vi "Get IO Names.vi"(8 "error in (no error)":errorcluster, 11 "Module in":refnum<class "Module.lvclass">) -> (0 "error out":errorcluster, 2 "IO Names":string[](array[string]), 3 "Module out":refnum<class "Module.lvclass">)   [LabVIEW 2019, in "Module.lvclass"]
uses:
  Module.lvclass
  Module.lvclass/Module.ctl
  Signal/Signal/Read IO Name.vi
  Signal/Signal/Signal.lvclass
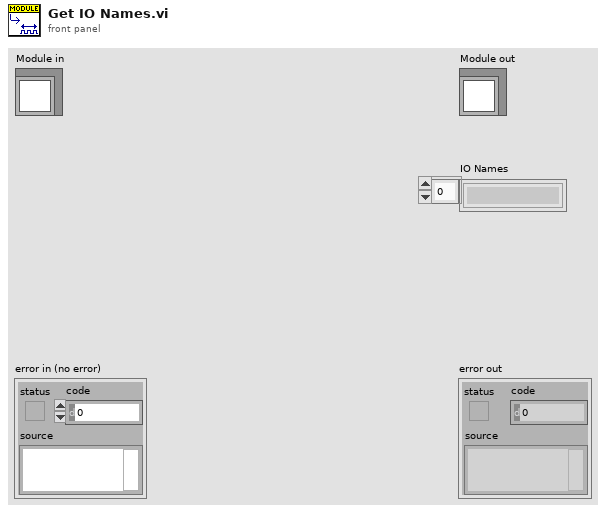
[diagram p1: front panel]
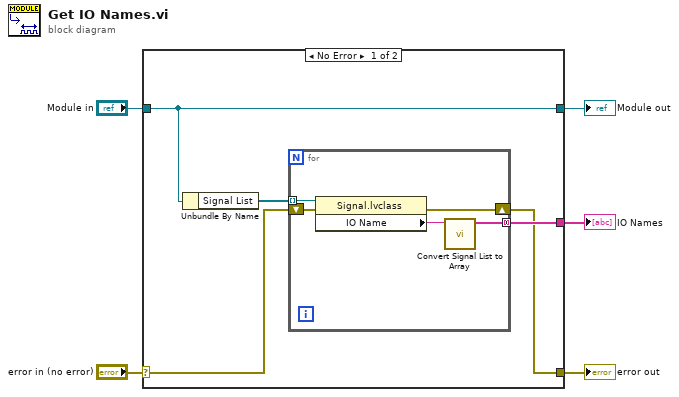
[diagram p0: block diagram]
diagram:
  n1 = case shown="No Error" "error in (no error)" {
    selector: "error in (no error)" -> [w7 w17]
    tunnel: [w6 w17] -> w4
    tunnel: [w10 w16] -> w2
    tunnel: "Module in" -> [w10 w16]
    tunnel: [w8 _] -> w1
    frame No Error {
      n2 = Unbundle By Name(w10) -> ("Signal List"=w9:refnum<class "Signal.lvclass">[])
      n3 = for {
        tunnel: w9 -> [w15] mode=indexing
        tunnel: [w11] -> w8 mode=concatenating
        shift-right: [w13] -> w6
        shift-left: w7 -> [w14]
        n4 = property class="Signal.lvclass"(reference=w15, error in=w14) -> (error out=w13:errorcluster, "IO Name"=w12:string)  [unwired: 1 out]
        n5 = call "Convert Signal List to Array.vi"("Signal List"=w12) -> ("Signal List"=w11:string[])  [unwired: 10 in]
      }
    }
    frame Error {
    }
  }
  "error out" <- w4
  "Module out" <- w2
  "IO Names" <- w1
